vi "auton single bo peep.vi"() -> ()   [LabVIEW 2014]
uses:
  <vilib>/Rock Robotics/WPI/Solenoid/WPI_SolenoidValue.ctl
  <vilib>/Rock Robotics/WPI/Solenoid/WPI_SolenoidGetEnum.vi
  Robot Global Data.vi
  <vilib>/Rock Robotics/WPI/Solenoid/WPI_SolenoidSetEnum.vi
  <vilib>/Rock Robotics/WPI/RobotDrive/WPI_RobotDriveGetSetRefNum.vi
  <vilib>/Rock Robotics/WPI/RobotDrive/WPI_RobotDriveMecanumDrive_Cartesian.vi
panel:
  out "Latched":bool
  out "Dump pressure valve state":T1
  out "Bo peep arm solenoid state":T1
  out "Bo Peep State":i8
  out "Wait for vacuum to attach timer":u32
  out "arm retract timer":u32=2000
  out "vacuum dump valve on dwell timer":u32=2000
  in  "arm retract time (ms)":u32=2000
  in  "vacuum dump valve on dwell (ms)":u32=2000
  in  "Waiting for Vacuum creep speed":dbl=0.25
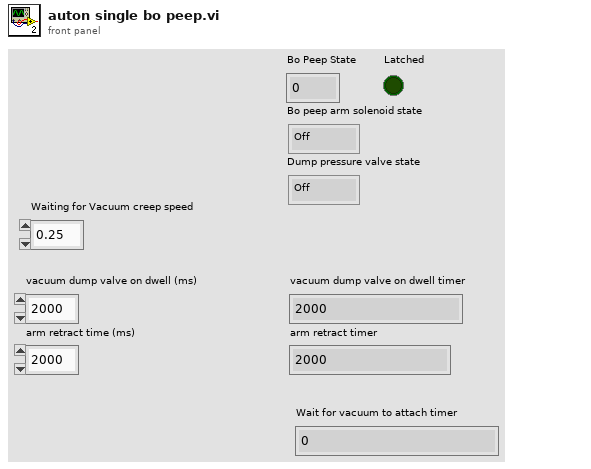
[diagram p1: front panel]
types:
  T1 = typedef "WPI_SolenoidValue.ctl" = enum16{"Off", "On", "Forward", "Reverse"}
  T2 = typedef "WPI_SolenoidDevRef.ctl" = cluster{"DevStatus":errorcluster, "Pneumatics Control Module":u8, "Forward Solenoid Channel":T3, "Reverse Solenoid Channel":T3}
  T3 = typedef "WPI_SolenoidChannel.ctl" = enum8{"Solenoid 0", "Solenoid 1", "Solenoid 2", "Solenoid 3", "Solenoid 4", "Solenoid 5", "Solenoid 6", "Solenoid 7", "Invalid"}
  T4 = typedef "WPI_RobotDriveDevRef.ctl" = cluster{"DevStatus":errorcluster, "Motors[]":T5[], "Square Inputs":bool, "Max Output":dbl}
  T5 = typedef "WPI_MotorControlDeviceRef.ctl" = cluster{"DeviceStatus":errorcluster, "Type":T6, "PWM":cluster{"Controller":T7, "PWM Channel":T8, "DeadBand":T9}, "CAN":cluster{"Device Number":u8, "Control Mode":T10, "Semaphore":T11, "Max Vout":dbl, "TalonSRX Control Mode":T12}, "Invert":bool, "TransformRef":T13, "InvTransformRef":T13}
  T6 = typedef "WPI_MotorControlType.ctl" = enum16{"PWM", "CAN", "CANTalonSRX"}
  T7 = typedef "FPGA_TypedefDigitalModule.ctl" = enum16{"Controller 1"}
  T8 = typedef "FPGA_DIOPWMChannel.ctl" = enum8{"PWM 0", "PWM 1", "PWM 2", "PWM 3", "PWM 4", "PWM 5", "PWM 6", "PWM 7", "PWM 8", "PWM 9", "PWM MXP 0", "PWM MXP 1", "PWM MXP 2", "PWM MXP 3", "PWM MXP 4", "PWM MXP 5", "PWM MXP 6", "PWM MXP 7", "PWM MXP 8", "PWM MXP 9", "Invalid"}
  T9 = typedef "WPI_PWMDeadband.ctl" = cluster{"Name":string, "maxPositivePwm":i32, "minPositivePwm":i32, "centerPwm":i32, "maxNegativePwm":i32, "minNegativePwm":i32, "angularRange":u16}
  T10 = typedef "WPI_CANJaguar_ControlMode.ctl" = enum8{"Percent VBus", "Current", "Speed", "Position", "Voltage"}
  T11 = typedef "Semaphore RefNum" = refnum<k1>
  T12 = typedef "WPI_CANTalonSRX_APIControlMode.ctl" = enum8{"Percent VBus", "Speed", "Position", "Slave", "Unchanged / Invalid"}
  T13 = typedef "WPI_PWMTransform_ConPane.ctl" = refnum<vi>
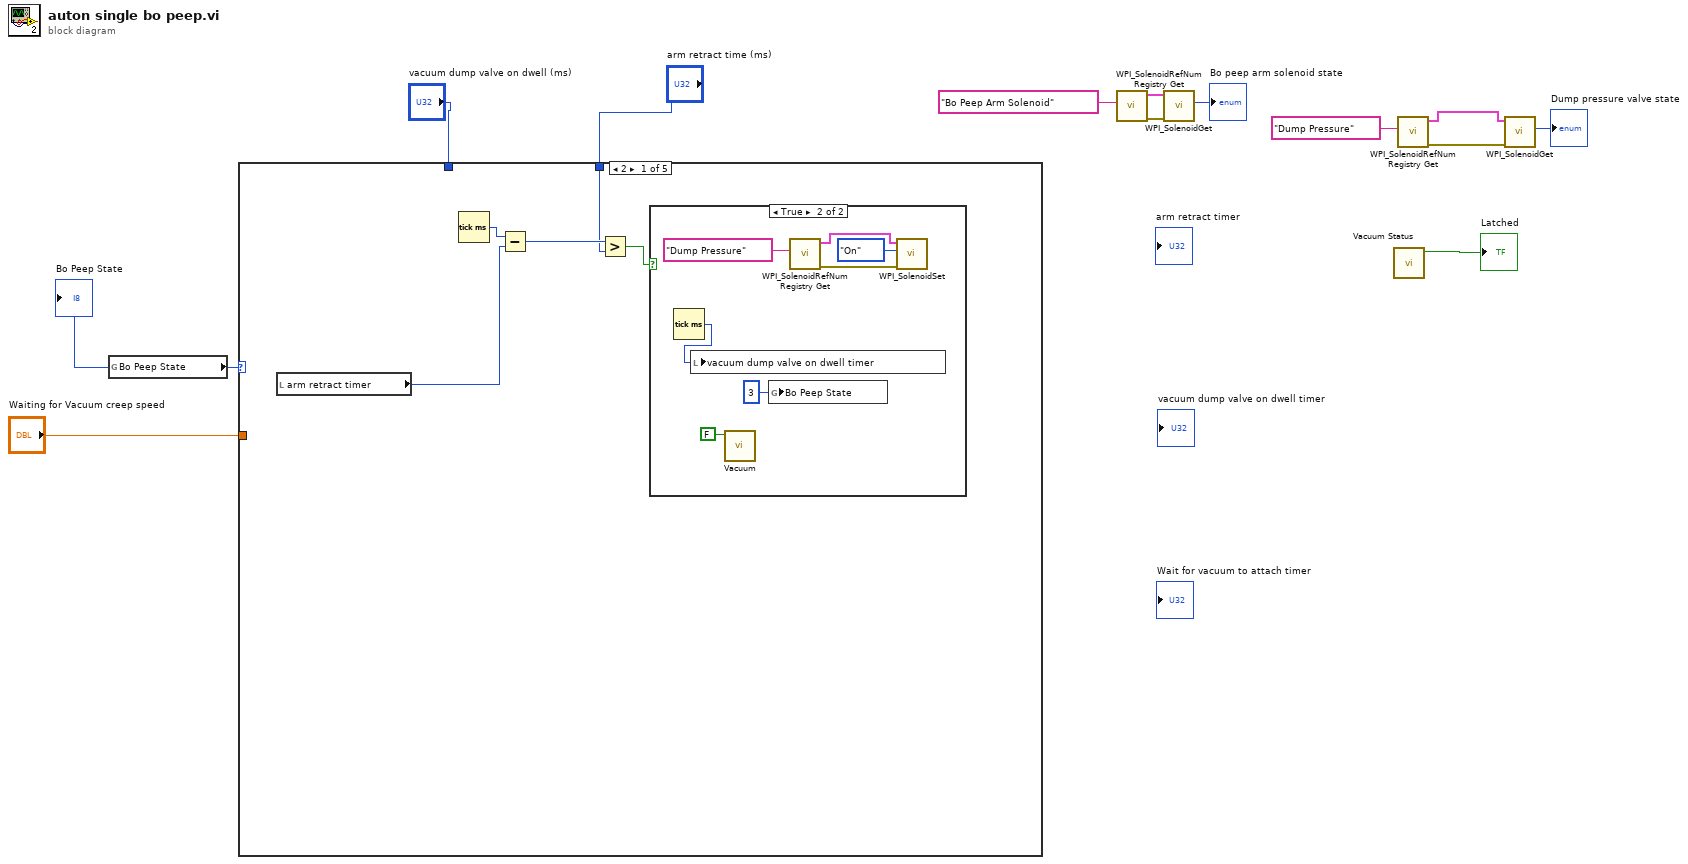
[diagram p0: block diagram]
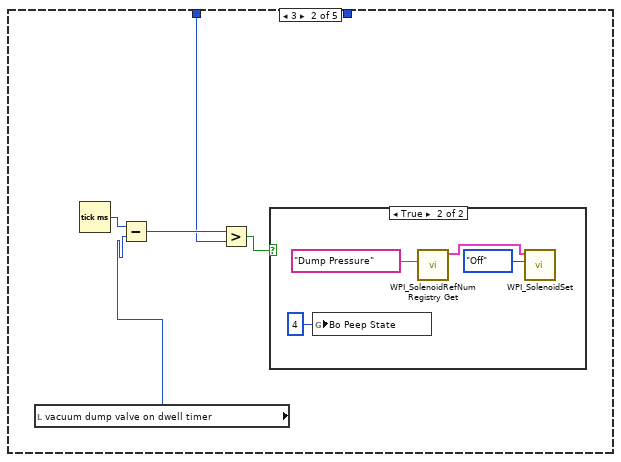
[diagram p3: hidden frame]
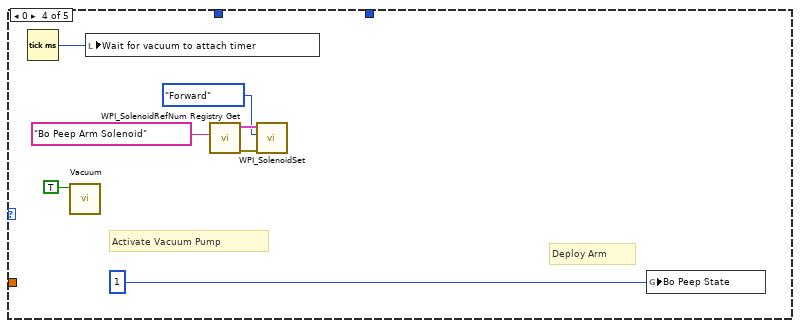
[diagram p6: hidden frame]
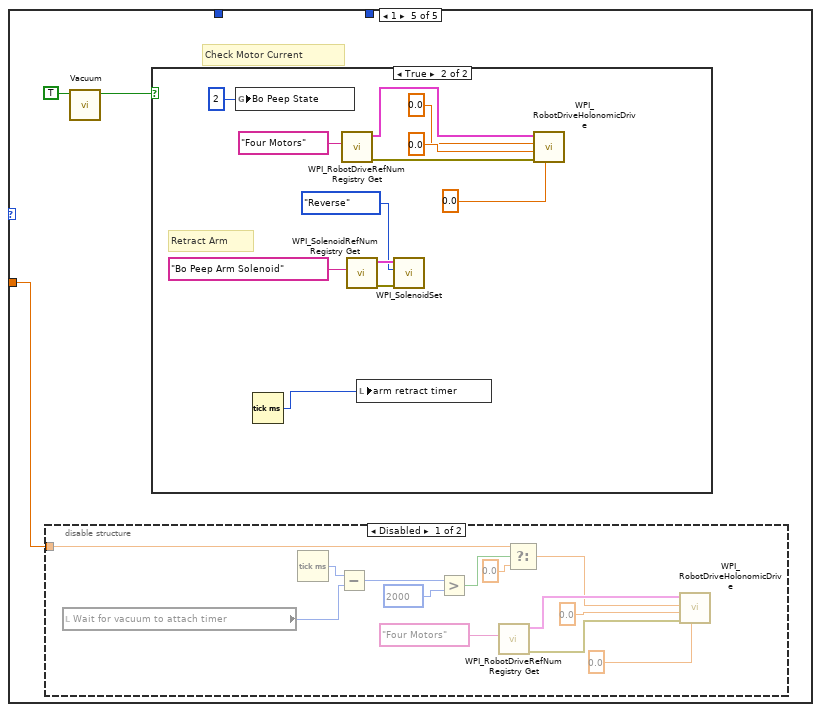
[diagram p7: hidden frame]
diagram:
  n1 = global read "Robot Global Data.vi" "Bo Peep State"() -> (w13:i8)
  "Bo Peep State" <- w13
  n2 = case shown="2" w13 {
    tunnel: "Waiting for Vacuum creep speed" -> [_ _ _ _ w42]
    tunnel: "vacuum dump valve on dwell (ms)" -> [_ w27 _ _ _]
    tunnel: "arm retract time (ms)" -> [w15 _ _ _ _]
    frame 2 {
      n3 = local read "arm retract timer"() -> (w14:u32)
      n4 = Tick Count (ms)() -> (millisecond timer value=w18:u32)
      n5 = Subtract(x=w18, y=w14) -> (x-y=w17:u32)
      n6 = Greater?(x=w17, y=w15) -> (0:w16:bool)
      n7 = case shown="True" w16 {
        frame False {
        }
        frame True {
          n8 = Tick Count (ms)() -> (millisecond timer value=w20:u32)
          n9 = local write "vacuum dump valve on dwell timer"(w20) -> ()
          n10 = call "Vacuum.vi"("Vacuum State"=FALSE) -> ()  [unwired: 9 in, 1 out]
          n11 = global write "Robot Global Data.vi" "Bo Peep State"(i8 3 ("Bo Peep State")) -> ()
          n12 = call <vilib>:"WPI_SolenoidRefNum Registry Get.vi"("refnum name"="Dump Pressure") -> ("error out"=w25:errorcluster, "SolenoidDevRef"=w19:T2)  [unwired: 9 in]
          n13 = call-poly <vilib>:"WPI_SolenoidSet.vi"("error in (no error)"=w25, "Value"=WPI_SolenoidValue."On", "SolenoidDevRef"=w19) -> ()  [unwired: 7 in, 2 out]
        }
      }
    }
    frame 3 {
      n14 = local read "vacuum dump valve on dwell timer"() -> (w26:u32)
      n15 = Tick Count (ms)() -> (millisecond timer value=w30:u32)
      n16 = Subtract(x=w30, y=w26) -> (x-y=w29:u32)
      n17 = Greater?(x=w29, y=w27) -> (0:w28:bool)
      n18 = case shown="True" w28 {
        frame False {
        }
        frame True {
          n19 = global write "Robot Global Data.vi" "Bo Peep State"(i8 4 ("Bo Peep State")) -> ()
          n20 = call <vilib>:"WPI_SolenoidRefNum Registry Get.vi"("refnum name"="Dump Pressure") -> ("SolenoidDevRef"=w33:T2)  [unwired: 9 in, 1 out]
          n21 = call-poly <vilib>:"WPI_SolenoidSet.vi"("Value"=WPI_SolenoidValue."Off", "SolenoidDevRef"=w33) -> ()  [unwired: 8 in, 2 out]
        }
      }
    }
    frame 4, Default {
    }
    frame 0 {
      # "Deploy Arm"
      # "Activate Vacuum Pump"
      n22 = Tick Count (ms)() -> (millisecond timer value=w35:u32)
      n23 = call "Vacuum.vi"("Vacuum State"=TRUE) -> ()  [unwired: 9 in, 1 out]
      n24 = local write "Wait for vacuum to attach timer"(w35) -> ()
      n25 = call <vilib>:"WPI_SolenoidRefNum Registry Get.vi"("refnum name"="Bo Peep Arm Solenoid") -> ("error out"=w39:errorcluster, "SolenoidDevRef"=w38:T2)  [unwired: 9 in]
      n26 = call-poly <vilib>:"WPI_SolenoidSet.vi"("error in (no error)"=w39, "Value"=WPI_SolenoidValue."Forward", "SolenoidDevRef"=w38) -> ()  [unwired: 7 in, 2 out]
      n27 = global write "Robot Global Data.vi" "Bo Peep State"(i8 1 ("Bo Peep State")) -> ()
    }
    frame 1 {
      # "Check Motor Current"
      n28 = disable-structure shown="Disabled" {
        disable-tunnel: w42 -> [w47 _]
        frame Disabled {
          n29 = local read "Wait for vacuum to attach timer"() -> (w45:u32)
          n30 = Tick Count (ms)() -> (millisecond timer value=w57:u32)
          n31 = Subtract(x=w57, y=w45) -> (x-y=w56:u32)
          n32 = Greater?(x=w56, y=u32 2000) -> (0:w49:bool)
          n33 = call <vilib>:"WPI_RobotDriveRefNum Registry Get.vi"("refnum name"="Four Motors") -> ("error out"=w53:errorcluster, "RobotDriveDevRef"=w50:T4)  [unwired: 9 in]
          n34 = Select(t=w47, s=w49, f=0.0) -> (s? t:f=w46:dbl)
          n35 = call-poly <vilib>:"WPI_RobotDriveHolonomicDrive.vi"("Rotation"=0.0, "error in (no error)"=w53, "Y"=0.0, "X"=w46, "RobotDriveDevRef"=w50) -> ()  [unwired: 4 in, 3 out]
        }
        frame Enabled {
        }
      }
      n36 = call "Vacuum.vi"("Vacuum State"=TRUE) -> ("Latched"=w44:bool)  [unwired: 9 in]
      n37 = case shown="True" w44 {
        frame False {
        }
        frame True {
          # "Retract Arm"
          n38 = global write "Robot Global Data.vi" "Bo Peep State"(i8 2 ("Bo Peep State")) -> ()
          n39 = Tick Count (ms)() -> (millisecond timer value=w58:u32)
          n40 = call <vilib>:"WPI_RobotDriveRefNum Registry Get.vi"("refnum name"="Four Motors") -> ("error out"=w67:errorcluster, "RobotDriveDevRef"=w64:T4)  [unwired: 9 in]
          n41 = call <vilib>:"WPI_SolenoidRefNum Registry Get.vi"("refnum name"="Bo Peep Arm Solenoid") -> ("error out"=w61:errorcluster, "SolenoidDevRef"=w60:T2)  [unwired: 9 in]
          n42 = local write "arm retract timer"(w58) -> ()
          n43 = call-poly <vilib>:"WPI_SolenoidSet.vi"("error in (no error)"=w61, "Value"=WPI_SolenoidValue."Reverse", "SolenoidDevRef"=w60) -> ()  [unwired: 7 in, 2 out]
          n44 = call-poly <vilib>:"WPI_RobotDriveHolonomicDrive.vi"("Rotation"=0.0, "error in (no error)"=w67, "Y"=0.0, "X"=0.0, "RobotDriveDevRef"=w64) -> ()  [unwired: 4 in, 3 out]
        }
      }
    }
  }
  n45 = call <vilib>:"WPI_SolenoidRefNum Registry Get.vi"("refnum name"="Bo Peep Arm Solenoid") -> ("error out"=w9:errorcluster, "SolenoidDevRef"=w8:T2)  [unwired: 9 in]
  n46 = call-poly <vilib>:"WPI_SolenoidGet.vi"("error in (no error)"=w9, "SolenoidDevRef"=w8) -> ("Value"=→"Bo peep arm solenoid state":T1)  [unwired: 7 in, 2 out]
  n47 = call "Vacuum Status.vi"() -> ("Latched"=→"Latched":bool)  [unwired: 10 in]
  n48 = call <vilib>:"WPI_SolenoidRefNum Registry Get.vi"("refnum name"="Dump Pressure") -> ("error out"=w5:errorcluster, "SolenoidDevRef"=w3:T2)  [unwired: 9 in]
  n49 = call-poly <vilib>:"WPI_SolenoidGet.vi"("error in (no error)"=w5, "SolenoidDevRef"=w3) -> ("Value"=→"Dump pressure valve state":T1)  [unwired: 7 in, 2 out]
